vi "ChoosePram.vi"(7 "Parameter Selection":u16(ring) items=["Neg Peak (V)", "Pos Peak  (V)", "Peak to Peak  (V)", "RMS  (V)", "Neg Peak Pressure (MPa)", "p.3 (MPa)", "Ipa (W/cm^2)", "Ipa.3 (W/cm^2)", "Ita (W/cm^2)", "Ita.3 (W/cm^2)"], 11 "Scan data":T1 {"Pulse Parameters"."pos peak pressure (MPa)" format="%.2f"; "axis 2 ticks" format="%.2f"; "axis 1 ticks" format="%.2f"; "step size" format="%.2f"; "axis2o" format="%.2f"; "axis1o" format="%.2f"; "scan data" format="%.2f"}) -> (3 "data out":dbl[][](array[numeric]) format="%.2f")   [LabVIEW 2022 SP3]
uses:
  <vilib>/Analysis/baseanly.llb/Mean (DBL).vi
  <vilib>/Analysis/5stat.llb/RMS (DBL).vi
  <vilib>/Analysis/NI_AALPro.lvlib
  <vilib>/Analysis/NI_AALBase.lvlib
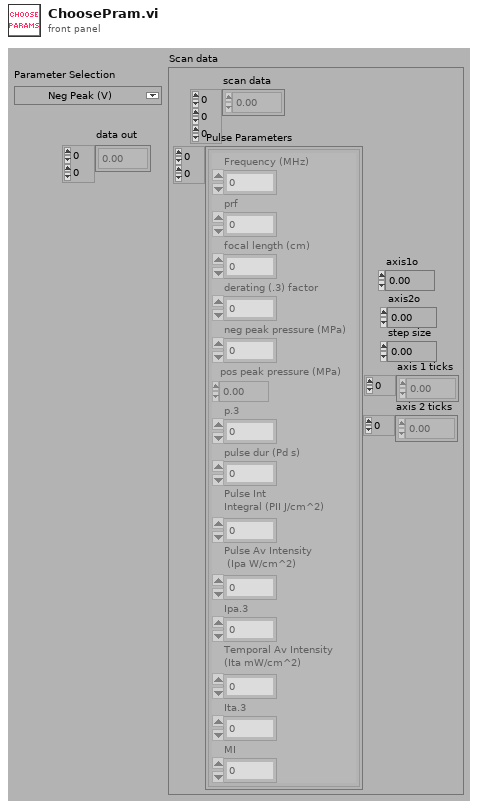
[diagram p1: front panel]
types:
  T1 = cluster{"scan data":dbl[][][], "Pulse Parameters":cluster{"Frequency (MHz)":dbl, "prf":dbl, "focal length (cm)":dbl, "derating (.3) factor":dbl, "neg peak pressure (MPa)":dbl, "pos peak pressure (MPa)":dbl, "p.3":dbl, "pulse dur (Pd s)":dbl, "Pulse Int \nIntegral (PII J/cm^2)":dbl, "Pulse Av Intensity\n (Ipa W/cm^2)":dbl, "Ipa.3":dbl, "Temporal Av Intensity \n(Ita mW/cm^2)":dbl, "Ita.3":dbl, "MI":dbl}[][], "axis1o":dbl, "axis2o":dbl, "step size":dbl, "axis 1 ticks":dbl[], "axis 2 ticks":dbl[]}
  T2 = cluster{"Frequency (MHz)":dbl, "prf":dbl, "focal length (cm)":dbl, "derating (.3) factor":dbl, "neg peak pressure (MPa)":dbl, "pos peak pressure (MPa)":dbl, "p.3":dbl, "pulse dur (Pd s)":dbl, "Pulse Int \nIntegral (PII J/cm^2)":dbl, "Pulse Av Intensity\n (Ipa W/cm^2)":dbl, "Ipa.3":dbl, "Temporal Av Intensity \n(Ita mW/cm^2)":dbl, "Ita.3":dbl, "MI":dbl}[][]
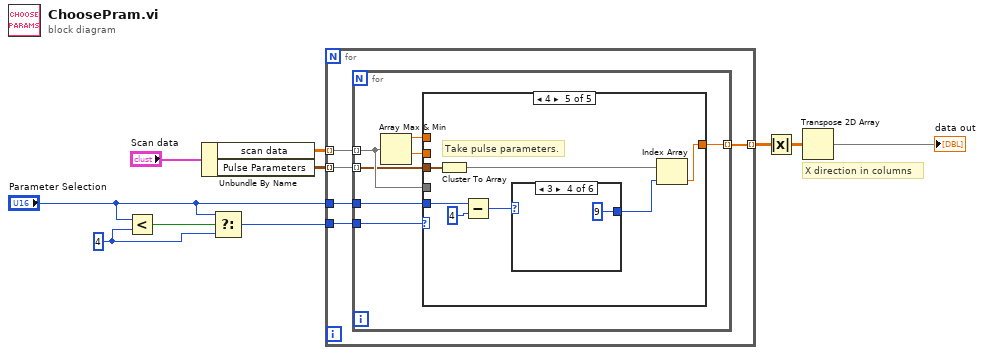
[diagram p0: block diagram]
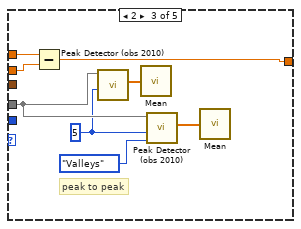
[diagram p4: hidden frame]
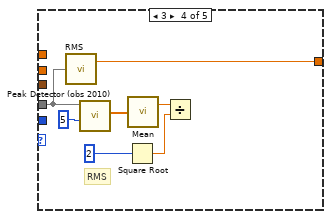
[diagram p5: hidden frame]
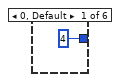
[diagram p6: hidden frame]
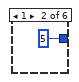
[diagram p7: hidden frame]
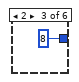
[diagram p8: hidden frame]
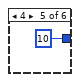
[diagram p9: hidden frame]
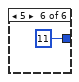
[diagram p10: hidden frame]
diagram:
  w9 = 4
  # "X direction in columns"
  n1 = Less?(x="Parameter Selection", y=w9) -> (x < y?=w10:bool)
  n2 = Unbundle By Name("Scan data") -> ("scan data"=w6:dbl[][][], "Pulse Parameters"=w1:T2)
  n3 = Select(t="Parameter Selection", s=w10, f=w9) -> (s? t:f=w8:i32)
  n4 = for {
    tunnel: w8 -> [w15]
    tunnel: [w14] -> w7 mode=indexing
    tunnel: w6 -> [w11] mode=indexing
    tunnel: "Parameter Selection" -> [w13]
    tunnel: w1 -> [w12] mode=indexing
    n5 = for {
      tunnel: w15 -> [w20]
      tunnel: [w19] -> w14 mode=indexing
      tunnel: w11 -> [w18] mode=indexing
      tunnel: w13 -> [w17]
      tunnel: w12 -> [w16] mode=indexing
      n6 = Array Max & Min(array=w18) -> (max value=w21:dbl, min value=w22:dbl)  [unwired: 2 out]
      n7 = case shown="4" w20 {
        tunnel: w22 -> [w23 _ w25 _ _]
        tunnel: w21 -> [_ w24 w26 _ _]
        tunnel: w18 -> [_ _ w32 w34 _]
        tunnel: [w23 w24 w27 w33 w40] -> w19
        tunnel: w17 -> [_ _ _ _ w44]
        tunnel: w16 -> [_ _ _ _ w43]
        frame 0, Default {
          # "neg peak"
        }
        frame 1 {
          # "pos peak"
        }
        frame 2 {
          w30 = 5 ("width")
          # "peak to peak"
          n8 = Subtract(x=w26, y=w25) -> (x-y=w27:dbl)
          n9 = call <vilib>:"Peak Detector (obs 2010).vi"("width"=w30, "X"=w32) -> ("Amplitudes"=w29:dbl[])  [unwired: 5 in, 4 out]
          n10 = call-poly <vilib>:"Mean.vi"("X"=w29) -> ()  [unwired: 2 out]
          n11 = call <vilib>:"Peak Detector (obs 2010).vi"("peaks/valleys"=enum32{"Peaks", "Valleys"}."Valleys", "width"=w30, "X"=w32) -> ("Amplitudes"=w28:dbl[])  [unwired: 4 in, 4 out]
          n12 = call-poly <vilib>:"Mean.vi"("X"=w28) -> ()  [unwired: 2 out]
        }
        frame 3 {
          # "RMS"
          n13 = call-poly <vilib>:"RMS.vi"("X"=w34) -> ("rms value"=w33:dbl)  [unwired: 1 out]
          n14 = call <vilib>:"Peak Detector (obs 2010).vi"("width"=5, "X"=w34) -> ("Amplitudes"=w39:dbl[])  [unwired: 5 in, 4 out]
          n15 = Square Root(x=2) -> (sqrt(x)=w35:dbl)
          n16 = call-poly <vilib>:"Mean.vi"("X"=w39) -> ("mean"=w37:dbl)  [unwired: 1 out]
          n17 = Divide(x=w37, y=w35) -> ()  [unwired: 1 out]
        }
        frame 4 {
          # "Take pulse parameters."
          n18 = Cluster To Array(cluster=w43) -> (array=w42:dbl[])
          n19 = Subtract(x=w44, y=4) -> (x-y=w45:i32)
          n20 = case shown="3" w45 {
            tunnel: [4 5 8 9 10 11] -> w41
            frame 0, Default {
            }
            frame 1 {
            }
            frame 2 {
            }
            frame 3 {
            }
            frame 4 {
            }
            frame 5 {
            }
          }
          n21 = Index Array(array=w42, index=w41) -> (element=w40:dbl)
        }
      }
    }
  }
  n22 = Absolute Value(x=w7) -> (abs(x)=w4:dbl[][])
  n23 = Transpose 2D Array(2D array=w4) -> (transposed array=→"data out":dbl[][])
